vi "nanocal -- nuclear schottky fit -- 2x2 -- V9.vi"() -> ()   [LabVIEW 2021] (continued)
\"τS\" -> 0.000000000000   ,  \"τN\" -> 0.000000000000   ,  \"τC\" -> 0.000000000000   ,  \"κ0\" -> 0.000000000000   ,  \"mm1\" -> 0.000000000000   ,  \"mm2\" -> 0.000000000000   ,  \"mm3\" -> 0.000000000000   ,  \"T\" -> 3.070000000000   ,  \"B\" -> 4.000000000000   ,  \"θ\" -> 0.000000000000   ,  \"Reoff\" -> 0.000000000000   ,  \"Imoff\" -> 0.000000000000   ,  \"στ1\" -> 0.000000000000   ,  \"στS\" -> 0.000000000000   ,  \"στN\" -> 0.000000000000    |>   , \n\"IDS0473_220531_RAW_cal__ref_\" ->   <|    \"ζ\" -> 0.018700689738   ,  \"τ1\" -> 0.039247142341   ,  \"τS\" -> 0.006094502124   ,  \"τN\" -> 0.000001379348   ,  \"τC\" -> 0.001765569741   ,  \"κ0\" -> 0.000000055137   ,  \"mm1\" -> 0.000025315301   ,  \"mm2\" -> 0.007948371438   ,  \"mm3\" -> 0.039248904003   ,  \"T\" -> 5.700000000000   ,  \"B\" -> 4.000000000000   ,  \"θ\" -> 0.000000000000   ,  \"Reoff\" -> -102040.816326530650   ,  \"Imoff\" -> 0.000000000000   ,  \"στ1\" -> 0.006123782667   ,  \"στS\" -> 0.001309533453   ,  \"στN\" -> 0.000000787923    |>   , \n\"IDS0473_220531_RAW_cal__sam_\" ->   <|    \"ζ\" -> 0.000000000000   ,  \"τ1\" -> 0.000000000000   ,  \"τS\" -> 0.000000000000   ,  \"τN\" -> 0.000000000000   ,  \"τC\" -> 0.000000000000   ,  \"κ0\" -> 0.000000000000   ,  \"mm1\" -> 0.000000000000   ,  \"mm2\" -> 0.000000000000   ,  \"mm3\" -> 0.000000000000   ,  \"T\" -> 5.700000000000   ,  \"B\" -> 4.000000000000   ,  \"θ\" -> 0.000000000000   ,  \"Reoff\" -> 0.000000000000   ,  \"Imoff\" -> 0.000000000000   ,  \"στ1\" -> 0.000000000000   ,  \"στS\" -> 0.000000000000   ,  \"στN\" -> 0.000000000000    |>   , \n\"IDS0477_220601_RAW_cal__ref_\" ->   <|    \"ζ\" -> 0.239805642697   ,  \"τ1\" -> 0.033790664831   ,  \"τS\" -> 0.059024379220   ,  \"τN\" -> 0.060427064379   ,  \"τC\" -> 0.000896937980   ,  \"κ0\" -> 0.000000000920   ,  \"mm1\" -> 0.000171776345   ,  \"mm2\" -> 0.014890032084   ,  \"mm3\" -> 0.167722368184   ,  \"T\" -> 0.200000000000   ,  \"B\" -> 10.000000000000   ,  \"θ\" -> 45.000000000000   ,  \"Reoff\" -> -36122448.979591839000   ,  \"Imoff\" -> 0.000000000000   ,  \"στ1\" -> 0.011907202865   ,  \"στS\" -> 0.006392080806   ,  \"στN\" -> 0.010956766376    |>   , \n\"IDS0477_220601_RAW_cal__sam_\" ->   <|    \"ζ\" -> 0.000000000000   ,  \"τ1\" -> 0.000000000000   ,  \"τS\" -> 0.000000000000   ,  \"τN\" -> 0.000000000000   ,  \"τC\" -> 0.000000000000   ,  \"κ0\" -> 0.000000000000   ,  \"mm1\" -> 0.000000000000   ,  \"mm2\" -> 0.000000000000   ,  \"mm3\" -> 0.000000000000   ,  \"T\" -> 0.200000000000   ,  \"B\" -> 10.000000000000   ,  \"θ\" -> 45.000000000000   ,  \"Reoff\" -> 0.000000000000   ,  \"Imoff\" -> 0.000000000000   ,  \"στ1\" -> 0.000000000000   ,  \"στS\" -> 0.000000000000   ,  \"στN\" -> 0.000000000000    |>   , \n\"IDS0478_220601_RAW_cal__ref_\" ->   <|    \"ζ\" -> 0.152803180528   ,  \"τ1\" -> 0.028187868792   ,  \"τS\" -> 0.047098340694   ,  \"τN\" -> 0.025207837056   ,  \"τC\" -> 0.000982024605   ,  \"κ0\" -> 0.000000001260   ,  \"mm1\" -> 0.000128146365   ,  \"mm2\" -> 0.016152622122   ,  \"mm3\" -> 0.096243916593   ,  \"T\" -> 0.250000000000   ,  \"B\" -> 10.000000000000   ,  \"θ\" -> 45.000000000000   ,  \"Reoff\" -> -18163265.306122452000   ,  \"Imoff\" -> 0.000000000000   ,  \"στ1\" -> 0.005041045857   ,  \"στS\" -> 0.001567344139   ,  \"στN\" -> 0.002277988599    |>   , \n\"IDS0478_220601_RAW_cal__sam_\" ->   <|    \"ζ\" -> 0.000000000000   ,  \"τ1\" -> 0.000000000000   ,  \"τS\" -> 0.000000000000   ,  \"τN\" -> 0.000000000000   ,  \"τC\" -> 0.000000000000   ,  \"κ0\" -> 0.000000000000   ,  \"mm1\" -> 0.000000000000   ,  \"mm2\" -> 0.000000000000   ,  \"mm3\" -> 0.000000000000   ,  \"T\" -> 0.250000000000   ,  \"B\" -> 10.000000000000   ,  \"θ\" -> 45.000000000000   ,  \"Reoff\" -> 0.000000000000   ,  \"Imoff\" -> 0.000000000000   ,  \"στ1\" -> 0.000000000000   ,  \"στS\" -> 0.000000000000   ,  \"στN\" -> 0.000000000000    |>   , \n\"IDS0479_220601_RAW_cal__ref_\" ->   <|    \"ζ\" -> 0.111193066205   ,  \"τ1\" -> 0.024122553376   ,  \"τS\" -> 0.042118651402   ,  \"τN\" -> 0.013651970206   ,  \"τC\" -> 0.001072327817   ,  \"κ0\" -> 0.000000001570   ,  \"mm1\" -> 0.000105128315   ,  \"mm2\" -> 0.016280391263   ,  \"mm3\" -> 0.070781289644   ,  \"T\" -> 0.300000000000   ,  \"B\" -> 10.000000000000   ,  \"θ\" -> 45.000000000000   ,  \"Reoff\" -> -10816326.530612245200   ,  \"Imoff\" -> 0.000000000000   ,  \"στ1\" -> 0.003531051170   ,  \"στS\" -> 0.000678989919   ,  \"στN\" -> 0.000877996668    |>   , \n\"IDS0479_220601_RAW_cal__sam_\" ->   <|    \"ζ\" -> 0.000000000000   ,  \"τ1\" -> 0.000000000000   ,  \"τS\" -> 0.000000000000   ,  \"τN\" -> 0.000000000000   ,  \"τC\" -> 0.000000000000   ,  \"κ0\" -> 0.000000000000   ,  \"mm1\" -> 0.000000000000   ,  \"mm2\" -> 0.000000000000   ,  \"mm3\" -> 0.000000000000   ,  \"T\" -> 0.300000000000   ,  \"B\" -> 10.000000000000   ,  \"θ\" -> 45.000000000000   ,  \"Reoff\" -> 0.000000000000   ,  \"Imoff\" -> 0.000000000000   ,  \"στ1\" -> 0.000000000000   ,  \"στS\" -> 0.000000000000   ,  \"στN\" -> 0.000000000000    |>   , \n\"IDS0480_220601_RAW_cal__ref_\" ->   <|    \"ζ\" -> 0.079231560459   ,  \"τ1\" -> 0.017107381840   ,  \"τS\" -> 0.036891145607   ,  \"τN\" -> 0.007202328301   ,  \"τC\" -> 0.001264563258   ,  \"κ0\" -> 0.000000002000   ,  \"mm1\" -> 0.000090175019   ,  \"mm2\" -> 0.013352548983   ,  \"mm3\" -> 0.052516289748   ,  \"T\" -> 0.360000000000   ,  \"B\" -> 10.000000000000   ,  \"θ\" -> 45.000000000000   ,  \"Reoff\" -> -6326530.612244904040   ,  \"Imoff\" -> 0.000000000000   ,  \"στ1\" -> 0.001933309697   ,  \"στS\" -> 0.000284795622   ,  \"στN\" -> 0.000344056722    |>   , \n\"IDS0480_220601_RAW_cal__sam_\" ->   <|    \"ζ\" -> 0.000000000000   ,  \"τ1\" -> 0.000000000000   ,  \"τS\" -> 0.000000000000   ,  \"τN\" -> 0.000000000000   ,  \"τC\" -> 0.000000000000   ,  \"κ0\" -> 0.000000000000   ,  \"mm1\" -> 0.000000000000   ,  \"mm2\" -> 0.000000000000   ,  \"mm3\" -> 0.000000000000   ,  \"T\" -> 0.360000000000   ,  \"B\" -> 10.000000000000   ,  \"θ\" -> 45.000000000000   ,  \"Reoff\" -> 0.000000000000   ,  \"Imoff\" -> 0.000000000000   ,  \"στ1\" -> 0.000000000000   ,  \"στS\" -> 0.000000000000   ,  \"στN\" -> 0.000000000000    |>   , \n\"IDS0481_220601_RAW_cal__ref_\" ->   <|    \"ζ\" -> 0.059346185114   ,  \"τ1\" -> 0.015969775027   ,  \"τS\" -> 0.034144098652   ,  \"τN\" -> 0.004294468384   ,  \"τC\" -> 0.001604549811   ,  \"κ0\" -> 0.000000002410   ,  \"mm1\" -> 0.000086265768   ,  \"mm2\" -> 0.013446939913   ,  \"mm3\" -> 0.044760868507   ,  \"T\" -> 0.420000000000   ,  \"B\" -> 10.000000000000   ,  \"θ\" -> 45.000000000000   ,  \"Reoff\" -> -3061224.489795923230   ,  \"Imoff\" -> 0.000000000000   ,  \"στ1\" -> 0.000907344416   ,  \"στS\" -> 0.000176030005   ,  \"στN\" -> 0.000148751487    |>   , \n\"IDS0481_220601_RAW_cal__sam_\" ->   <|    \"ζ\" -> 0.000000000000   ,  \"τ1\" -> 0.000000000000   ,  \"τS\" -> 0.000000000000   ,  \"τN\" -> 0.000000000000   ,  \"τC\" -> 0.000000000000   ,  \"κ0\" -> 0.000000000000   ,  \"mm1\" -> 0.000000000000   ,  \"mm2\" -> 0.000000000000   ,  \"mm3\" -> 0.000000000000   ,  \"T\" -> 0.420000000000   ,  \"B\" -> 10.000000000000   ,  \"θ\" -> 45.000000000000   ,  \"Reoff\" -> 0.000000000000   ,  \"Imoff\" -> 0.000000000000   ,  \"στ1\" -> 0.000000000000   ,  \"στS\" -> 0.000000000000   ,  \"στN\" -> 0.000000000000    |>   , \n\"IDS0482_220601_RAW_cal__ref_\" ->   <|    \"ζ\" -> 0.043142553496   ,  \"τ1\" -> 0.014499389185   ,  \"τS\" -> 0.030371945733   ,  \"τN\" -> 0.002402650316   ,  \"τC\" -> 0.001877907190   ,  \"κ0\" -> 0.000000003100   ,  \"mm1\" -> 0.000073480289   ,  \"mm2\" -> 0.012924539137   ,  \"mm3\" -> 0.037567852762   ,  \"T\" -> 0.520000000000   ,  \"B\" -> 10.000000000000   ,  \"θ\" -> 45.000000000000   ,  \"Reoff\" -> -1836734.693877555430   ,  \"Imoff\" -> 0.000000000000   ,  \"στ1\" -> 0.000488095502   ,  \"στS\" -> 0.000097405917   ,  \"στN\" -> 0.000051506778    |>   , \n\"IDS0482_220601_RAW_cal__sam_\" ->   <|    \"ζ\" -> 0.000000000000   ,  \"τ1\" -> 0.000000000000   ,  \"τS\" -> 0.000000000000   ,  \"τN\" -> 0.000000000000   ,  \"τC\" -> 0.000000000000   ,  \"κ0\" -> 0.000000000000   ,  \"mm1\" -> 0.000000000000   ,  \"mm2\" -> 0.000000000000   ,  \"mm3\" -> 0.000000000000   ,  \"T\" -> 0.520000000000   ,  \"B\" -> 10.000000000000   ,  \"θ\" -> 45.000000000000   ,  \"Reoff\" -> 0.000000000000   ,  \"Imoff\" -> 0.000000000000   ,  \"στ1\" -> 0.000000000000   ,  \"στS\" -> 0.000000000000   ,  \"στN\" -> 0.000000000000    |>   , \n\"IDS0483_220601_RAW_cal__ref_\" ->   <|    \"ζ\" -> 0.037957534412   ,  \"τ1\" -> 0.013025982486   ,  \"τS\" -> 0.027861955043   ,  \"τN\" -> 0.001482537125   ,  \"τC\" -> 0.001562153050   ,  \"κ0\" -> 0.000000003750   ,  \"mm1\" -> 0.000054295490   ,  \"mm2\" -> 0.012021211304   ,  \"mm3\" -> 0.032970965481   ,  \"T\" -> 0.620000000000   ,  \"B\" -> 10.000000000000   ,  \"θ\" -> 45.000000000000   ,  \"Reoff\" -> -2489795.918367348610   ,  \"Imoff\" -> 0.000000000000   ,  \"στ1\" -> 0.000872811735   ,  \"στS\" -> 0.000114206450   ,  \"στN\" -> 0.000055407234    |>   , \n\"IDS0483_220601_RAW_cal__sam_\" ->   <|    \"ζ\" -> 0.000000000000   ,  \"τ1\" -> 0.000000000000   ,  \"τS\" -> 0.000000000000   ,  \"τN\" -> 0.000000000000   ,  \"τC\" -> 0.000000000000   ,  \"κ0\" -> 0.000000000000   ,  \"mm1\" -> 0.000000000000   ,  \"mm2\" -> 0.000000000000   ,  \"mm3\" -> 0.000000000000   ,  \"T\" -> 0.620000000000   ,  \"B\" -> 10.000000000000   ,  \"θ\" -> 45.000000000000   ,  \"Reoff\" -> 0.000000000000   ,  \"Imoff\" -> 0.000000000000   ,  \"στ1\" -> 0.000000000000   ,  \"στS\" -> 0.000000000000   ,  \"στN\" -> 0.000000000000    |>   , \n\"IDS0484_220601_RAW_cal__ref_\" ->   <|    \"ζ\" -> 0.026779879048   ,  \"τ1\" -> 0.012724854717   ,  \"τS\" -> 0.023406495826   ,  \"τN\" -> 0.000845574693   ,  \"τC\" -> 0.002190018434   ,  \"κ0\" -> 0.000000005114   ,  \"mm1\" -> 0.000052452848   ,  \"mm2\" -> 0.011990951083   ,  \"mm3\" -> 0.027773007254   ,  \"T\" -> 0.820000000000   ,  \"B\" -> 10.000000000000   ,  \"θ\" -> 45.000000000000   ,  \"Reoff\" -> -1020408.163265310230   ,  \"Imoff\" -> 0.000000000000   ,  \"στ1\" -> 0.000585844678   ,  \"στS\" -> 0.000123901377   ,  \"στN\" -> 0.000022627070    |>   , \n\"IDS0484_220601_RAW_cal__sam_\" ->   <|    \"ζ\" -> 0.000000000000   ,  \"τ1\" -> 0.000000000000   ,  \"τS\" -> 0.000000000000   ,  \"τN\" -> 0.000000000000   ,  \"τC\" -> 0.000000000000   ,  \"κ0\" -> 0.000000000000   ,  \"mm1\" -> 0.000000000000   ,  \"mm2\" -> 0.000000000000   ,  \"mm3\" -> 0.000000000000   ,  \"T\" -> 0.820000000000   ,  \"B\" -> 10.000000000000   ,  \"θ\" -> 45.000000000000   ,  \"Reoff\" -> 0.000000000000   ,  \"Imoff\" -> 0.000000000000   ,  \"στ1\" -> 0.000000000000   ,  \"στS\" -> 0.000000000000   ,  \"στN\" -> 0.000000000000    |>   , \n\"IDS0485_220601_RAW_cal__ref_\" ->   <|    \"ζ\" -> 0.326622885443   ,  \"τ1\" -> 0.044212332753   ,  \"τS\" -> 0.078119393187   ,  \"τN\" -> 0.109436103453   ,  \"τC\" -> 0.000856629079   ,  \"κ0\" -> 0.000000000725   ,  \"mm1\" -> 0.000209590105   ,  \"mm2\" -> 0.016643396508   ,  \"mm3\" -> 0.277031389353   ,  \"T\" -> 0.170000000000   ,  \"B\" -> 10.000000000000   ,  \"θ\" -> 45.000000000000   ,  \"Reoff\" -> -62040816.326530613000   ,  \"Imoff\" -> 0.000000000000   ,  \"στ1\" -> 0.024054965225   ,  \"στS\" -> 0.017110063636   ,  \"στN\" -> 0.032486922745    |>   , \n\"IDS0485_220601_RAW_cal__sam_\" ->   <|    \"ζ\" -> 0.000000000000   ,  \"τ1\" -> 0.000000000000   ,  \"τS\" -> 0.000000000000   ,  \"τN\" -> 0.000000000000   ,  \"τC\" -> 0.000000000000   ,  \"κ0\" -> 0.000000000000   ,  \"mm1\" -> 0.000000000000   ,  \"mm2\" -> 0.000000000000   ,  \"mm3\" -> 0.000000000000   ,  \"T\" -> 0.170000000000   ,  \"B\" -> 10.000000000000   ,  \"θ\" -> 45.000000000000   ,  \"Reoff\" -> 0.000000000000   ,  \"Imoff\" -> 0.000000000000   ,  \"στ1\" -> 0.000000000000   ,  \"στS\" -> 0.000000000000   ,  \"στN\" -> 0.000000000000    |>   , \n\"IDS0486_220602_RAW_cal__ref_\" ->   <|    \"ζ\" -> 0.647357967210   ,  \"τ1\" -> 0.057848718155   ,  \"τS\" -> 0.135216834392   ,  \"τN\" -> 0.439833290844   ,  \"τC\" -> 0.000803496040   ,  \"κ0\" -> 0.000000000457   ,  \"mm1\" -> 0.000315044381   ,  \"mm2\" -> 0.013010354662   ,  \"mm3\" -> 0.992640220504   ,  \"T\" -> 0.120000000000   ,  \"B\" -> 10.000000000000   ,  \"θ\" -> 45.000000000000   ,  \"Reoff\" -> -171836734.693877578000   ,  \"Imoff\" -> 0.000000000000   ,  \"στ1\" -> 0.042149570105   ,  \"στS\" -> 0.062954836972   ,  \"στN\" -> 0.160749966190    |>   , \n\"IDS0486_220602_RAW_cal__sam_\" ->   <|    \"ζ\" -> 0.000000000000   ,  \"τ1\" -> 0.000000000000   ,  \"τS\" -> 0.000000000000   ,  \"τN\" -> 0.000000000000   ,  \"τC\" -> 0.000000000000   ,  \"κ0\" -> 0.000000000000   ,  \"mm1\" -> 0.000000000000   ,  \"mm2\" -> 0.000000000000   ,  \"mm3\" -> 0.000000000000   ,  \"T\" -> 0.120000000000   ,  \"B\" -> 10.000000000000   ,  \"θ\" -> 45.000000000000   ,  \"Reoff\" -> 0.000000000000   ,  \"Imoff\" -> 0.000000000000   ,  \"στ1\" -> 0.000000000000   ,  \"στS\" -> 0.000000000000   ,  \"στN\" -> 0.000000000000    |>   , \n\"IDS0487_220602_RAW_cal__ref_\" ->   <|    \"ζ\" -> 0.413977366659   ,  \"τ1\" -> 0.044491025512   ,  \"τS\" -> 0.091456784931   ,  \"τN\" -> 0.162770283044   ,  \"τC\" -> 0.000783758784   ,  \"κ0\" -> 0.000000000637   ,  \"mm1\" -> 0.000228474902   ,  \"mm2\" -> 0.014828264072   ,  \"mm3\" -> 0.389689365431   ,  \"T\" -> 0.150000000000   ,  \"B\" -> 10.000000000000   ,  \"θ\" -> 45.000000000000   ,  \"Reoff\" -> -87632653.061224490400   ,  \"Imoff\" -> 0.000000000000   ,  \"στ1\" -> 0.020687994730   ,  \"στS\" -> 0.021344943576   ,  \"στN\" -> 0.040787910782    |>   , \n\"IDS0487_220602_RAW_cal__sam_\" ->   <|    \"ζ\" -> 0.000000000000   ,  \"τ1\" -> 0.000000000000   ,  \"τS\" -> 0.000000000000   ,  \"τN\" -> 0.000000000000   ,  \"τC\" -> 0.000000000000   ,  \"κ0\" -> 0.000000000000   ,  \"mm1\" -> 0.000000000000   ,  \"mm2\" -> 0.000000000000   ,  \"mm3\" -> 0.000000000000   ,  \"T\" -> 0.150000000000   ,  \"B\" -> 10.000000000000   ,  \"θ\" -> 45.000000000000   ,  \"Reoff\" -> 0.000000000000   ,  \"Imoff\" -> 0.000000000000   ,  \"στ1\" -> 0.000000000000   ,  \"στS\" -> 0.000000000000   ,  \"στN\" -> 0.000000000000    |>   , \n\"IDS0488_220602_RAW_cal__ref_\" ->   <|    \"ζ\" -> 0.022173506919   ,  \"τ1\" -> 0.011885040231   ,  \"τS\" -> 0.019213986471   ,  \"τN\" -> 0.000342476634   ,  \"τC\" -> 0.002250605678   ,  \"κ0\" -> 0.000000007250   ,  \"mm1\" -> 0.000043889604   ,  \"mm2\" -> 0.011496376729   ,  \"mm3\" -> 0.022585478052   ,  \"T\" -> 1.120000000000   ,  \"B\" -> 10.000000000000   ,  \"θ\" -> 45.000000000000   ,  \"Reoff\" -> -775510.204081632196   ,  \"Imoff\" -> 0.000000000000   ,  \"στ1\" -> 0.000592033773   ,  \"στS\" -> 0.000127596201   ,  \"στN\" -> 0.000006161863    |>   , \n\"IDS0488_220602_RAW_cal__sam_\" ->   <|    \"ζ\" -> 0.000000000000   ,  \"τ1\" -> 0.000000000000   ,  \"τS\" -> 0.000000000000   ,  \"τN\" -> 0.000000000000   ,  \"τC\" -> 0.000000000000   ,  \"κ0\" -> 0.000000000000   ,  \"mm1\" -> 0.000000000000   ,  \"mm2\" -> 0.000000000000   ,  \"mm3\" -> 0.000000000000   ,  \"T\" -> 1.120000000000   ,  \"B\" -> 10.000000000000   ,  \"θ\" -> 45.000000000000   ,  \"Reoff\" -> 0.000000000000   ,  \"Imoff\" -> 0.000000000000   ,  \"στ1\" -> 0.000000000000   ,  \"στS\" -> 0.000000000000   ,  \"στN\" -> 0.000000000000    |>   , \n\"IDS0489_220602_RAW_cal__ref_\" ->   <|    \"ζ\" -> 0.017747577510   ,  \"τ1\" -> 0.012094843134   ,  \"τS\" -> 0.012989013001   ,  \"τN\" -> 0.000085603032   ,  \"τC\" -> 0.003089605627   ,  \"κ0\" -> 0.000000012681   ,  \"mm1\" -> 0.000043787767   ,  \"mm2\" -> 0.011860461021   ,  \"mm3\" -> 0.016586858767   ,  \"T\" -> 1.900000000000   ,  \"B\" -> 10.000000000000   ,  \"θ\" -> 45.000000000000   ,  \"Reoff\" -> -285714.285714283585   ,  \"Imoff\" -> 0.000000000000   ,  \"στ1\" -> 0.000492222129   ,  \"στS\" -> 0.000068169784   ,  \"στN\" -> 0.000002379689    |>   , \n\"IDS0489_220602_RAW_cal__sam_\" ->   <|    \"ζ\" -> 0.000000000000   ,  \"τ1\" -> 0.000000000000   ,  \"τS\" -> 0.000000000000   ,  \"τN\" -> 0.000000000000   ,  \"τC\" -> 0.000000000000   ,  \"κ0\" -> 0.000000000000   ,  \"mm1\" -> 0.000000000000   ,  \"mm2\" -> 0.000000000000   ,  \"mm3\" -> 0.000000000000   ,  \"T\" -> 1.900000000000   ,  \"B\" -> 10.000000000000   ,  \"θ\" -> 45.000000000000   ,  \"Reoff\" -> 0.000000000000   ,  \"Imoff\" -> 0.000000000000   ,  \"στ1\" -> 0.000000000000   ,  \"στS\" -> 0.000000000000   ,  \"στN\" -> 0.000000000000    |>   , \n\"IDS0490_220602_RAW_cal__ref_\" ->   <|    \"ζ\" -> 0.017719366864   ,  \"τ1\" -> 0.012304843107   ,  \"τS\" -> 0.009230373075   ,  \"τN\" -> 0.000023645241   ,  \"τC\" -> 0.002722388049   ,  \"κ0\" -> 0.000000022572   ,  \"mm1\" -> 0.000036861190   ,  \"mm2\" -> 0.011651022890   ,  \"mm3\" -> 0.012757340738   ,  \"T\" -> 3.100000000000   ,  \"B\" -> 10.000000000000   ,  \"θ\" -> 45.000000000000   ,  \"Reoff\" -> -204081.632653061300   ,  \"Imoff\" -> 0.000000000000   ,  \"στ1\" -> 0.000238275245   ,  \"στS\" -> 0.000083164391   ,  \"στN\" -> 0.000000428704    |>   , \n\"IDS0490_220602_RAW_cal__sam_\" ->   <|    \"ζ\" -> 0.000000000000   ,  \"τ1\" -> 0.000000000000   ,  \"τS\" -> 0.000000000000   ,  \"τN\" -> 0.000000000000   ,  \"τC\" -> 0.000000000000   ,  \"κ0\" -> 0.000000000000   ,  \"mm1\" -> 0.000000000000   ,  \"mm2\" -> 0.000000000000   ,  \"mm3\" -> 0.000000000000   ,  \"T\" -> 3.100000000000   ,  \"B\" -> 10.000000000000   ,  \"θ\" -> 45.000000000000   ,  \"Reoff\" -> 0.000000000000   ,  \"Imoff\" -> 0.000000000000   ,  \"στ1\" -> 0.000000000000   ,  \"στS\" -> 0.000000000000   ,  \"στN\" -> 0.000000000000    |>   , \n\"IDS0491_220602_RAW_cal__ref_\" ->   <|    \"ζ\" -> 0.018539000460   ,  \"τ1\" -> 0.012513981678   ,  \"τS\" -> 0.005770088680   ,  \"τN\" -> 0.000004734838   ,  \"τC\" -> 0.002222689414   ,  \"κ0\" -> 0.000000055495   ,  \"mm1\" -> 0.000029461735   ,  \"mm2\" -> 0.008061568111   ,  \"mm3\" -> 0.012527524219   ,  \"T\" -> 5.700000000000   ,  \"B\" -> 10.000000000000   ,  \"θ\" -> 45.000000000000   ,  \"Reoff\" -> -69387.755102040828   ,  \"Imoff\" -> 0.000000000000   ,  \"στ1\" -> 0.001996888534   ,  \"στS\" -> 0.001027587268   ,  \"στN\" -> 0.000002006873    |>   , \n\"IDS0491_220602_RAW_cal__sam_\" ->   <|    \"ζ\" -> 0.000000000000   ,  \"τ1\" -> 0.000000000000   ,  \"τS\" -> 0.000000000000   ,  \"τN\" -> 0.000000000000   ,  \"τC\" -> 0.000000000000   ,  \"κ0\" -> 0.000000000000   ,  \"mm1\" -> 0.000000000000   ,  \"mm2\" -> 0.000000000000   ,  \"mm3\" -> 0.000000000000   ,  \"T\" -> 5.700000000000   ,  \"B\" -> 10.000000000000   ,  \"θ\" -> 45.000000000000   ,  \"Reoff\" -> 0.000000000000   ,  \"Imoff\" -> 0.000000000000   ,  \"στ1\" -> 0.000000000000   ,  \"στS\" -> 0.000000000000   ,  \"στN\" -> 0.000000000000    |>   , \n\"IDS0493_220602_RAW_cal__ref_\" ->   <|    \"ζ\" -> 0.240316518824   ,  \"τ1\" -> 0.030134211391   ,  \"τS\" -> 0.077333506670   ,  \"τN\" -> 0.032228870252   ,  \"τC\" -> 0.000888040946   ,  \"κ0\" -> 0.000000000940   ,  \"mm1\" -> 0.000170781534   ,  \"mm2\" -> 0.019820439561   ,  \"mm3\" -> 0.146923057180   ,  \"T\" -> 0.200000000000   ,  \"B\" -> 8.000000000000   ,  \"θ\" -> 45.000000000000   ,  \"Reoff\" -> -33763265.306122481800   ,  \"Imoff\" -> 0.000000000000   ,  \"στ1\" -> 0.022409669919   ,  \"στS\" -> 0.010038141046   ,  \"στN\" -> 0.010969652299    |>   , \n\"IDS0493_220602_RAW_cal__sam_\" ->   <|    \"ζ\" -> 0.000000000000   ,  \"τ1\" -> 0.000000000000   ,  \"τS\" -> 0.000000000000   ,  \"τN\" -> 0.000000000000   ,  \"τC\" -> 0.000000000000   ,  \"κ0\" -> 0.000000000000   ,  \"mm1\" -> 0.000000000000   ,  \"mm2\" -> 0.000000000000   ,  \"mm3\" -> 0.000000000000   ,  \"T\" -> 0.200000000000   ,  \"B\" -> 8.000000000000   ,  \"θ\" -> 45.000000000000   ,  \"Reoff\" -> 0.000000000000   ,  \"Imoff\" -> 0.000000000000   ,  \"στ1\" -> 0.000000000000   ,  \"στS\" -> 0.000000000000   ,  \"στN\" -> 0.000000000000    |>   , \n\"IDS0494_220602_RAW_cal__ref_\" ->   <|    \"ζ\" -> 0.158252879790   ,  \"τ1\" -> 0.024827950008   ,  \"τS\" -> 0.060146890842   ,  \"τN\" -> 0.015050943013   ,  \"τC\" -> 0.000951750255   ,  \"κ0\" -> 0.000000001243   ,  \"mm1\" -> 0.000128517617   ,  \"mm2\" -> 0.018585917114   ,  \"mm3\" -> 0.094163373149   ,  \"T\" -> 0.250000000000   ,  \"B\" -> 8.000000000000   ,  \"θ\" -> 45.000000000000   ,  \"Reoff\" -> -20024489.795918367800   ,  \"Imoff\" -> 0.000000000000   ,  \"στ1\" -> 0.008614865267   ,  \"στS\" -> 0.002364789587   ,  \"στN\" -> 0.002490160339    |>   , \n\"IDS0494_220602_RAW_cal__sam_\" ->   <|    \"ζ\" -> 0.000000000000   ,  \"τ1\" -> 0.000000000000   ,  \"τS\" -> 0.000000000000   ,  \"τN\" -> 0.000000000000   ,  \"τC\" -> 0.000000000000   ,  \"κ0\" -> 0.000000000000   ,  \"mm1\" -> 0.000000000000   ,  \"mm2\" -> 0.000000000000   ,  \"mm3\" -> 0.000000000000   ,  \"T\" -> 0.250000000000   ,  \"B\" -> 8.000000000000   ,  \"θ\" -> 45.000000000000   ,  \"Reoff\" -> 0.000000000000   ,  \"Imoff\" -> 0.000000000000   ,  \"στ1\" -> 0.000000000000   ,  \"στS\" -> 0.000000000000   ,  \"στN\" -> 0.000000000000    |>   , \n\"IDS0495_220602_RAW_cal__ref_\" ->   <|    \"ζ\" -> 0.620326639374   ,  \"τ1\" -> 0.043464597459   ,  \"τS\" -> 0.134106398601   ,  \"τN\" -> 0.331630286291   ,  \"τC\" -> 0.000791545838   ,  \"κ0\" -> 0.000000000449   ,  \"mm1\" -> 0.000302343125   ,  \"mm2\" -> 0.012035033998   ,  \"mm3\" -> 0.786564323638   ,  \"T\" -> 0.120000000000   ,  \"B\" -> 8.000000000000   ,  \"θ\" -> 45.000000000000   ,  \"Reoff\" -> -197355102.040816367000   ,  \"Imoff\" -> 0.000000000000   ,  \"στ1\" -> 0.040479747535   ,  \"στS\" -> 0.067583774677   ,  \"στN\" -> 0.126300079114    |>   , \n\"IDS0495_220602_RAW_cal__sam_\" ->   <|    \"ζ\" -> 0.000000000000   ,  \"τ1\" -> 0.000000000000   ,  \"τS\" -> 0.000000000000   ,  \"τN\" -> 0.000000000000   ,  \"τC\" -> 0.000000000000   ,  \"κ0\" -> 0.000000000000   ,  \"mm1\" -> 0.000000000000   ,  \"mm2\" -> 0.000000000000   ,  \"mm3\" -> 0.000000000000   ,  \"T\" -> 0.120000000000   ,  \"B\" -> 8.000000000000   ,  \"θ\" -> 45.000000000000   ,  \"Reoff\" -> 0.000000000000   ,  \"Imoff\" -> 0.000000000000   ,  \"στ1\" -> 0.000000000000   ,  \"στS\" -> 0.000000000000   ,  \"στN\" -> 0.000000000000    |>   , \n\"IDS0496_220602_RAW_cal__ref_\" ->   <|    \"ζ\" -> 0.427468854343   ,  \"τ1\" -> 0.039705721457   ,  \"τS\" -> 0.111520336177   ,  \"τN\" -> 0.118737423491   ,  \"τC\" -> 0.000757643682   ,  \"κ0\" -> 0.000000000613   ,  \"mm1\" -> 0.000226123834   ,  \"mm2\" -> 0.018076446652   ,  \"mm3\" -> 0.350846575050   ,  \"T\" -> 0.150000000000   ,  \"B\" -> 8.000000000000   ,  \"θ\" -> 45.000000000000   ,  \"Reoff\" -> -103289795.918367386000   ,  \"Imoff\" -> 0.000000000000   ,  \"στ1\" -> 0.024554050195   ,  \"στS\" -> 0.027075430846   ,  \"στN\" -> 0.033199054106    |>   , \n\"IDS0496_220602_RAW_cal__sam_\" ->   <|    \"ζ\" -> 0.000000000000   ,  \"τ1\" -> 0.000000000000   ,  \"τS\" -> 0.000000000000   ,  \"τN\" -> 0.000000000000   ,  \"τC\" -> 0.000000000000   ,  \"κ0\" -> 0.000000000000   ,  \"mm1\" -> 0.000000000000   ,  \"mm2\" -> 0.000000000000   ,  \"mm3\" -> 0.000000000000   ,  \"T\" -> 0.150000000000   ,  \"B\" -> 8.000000000000   ,  \"θ\" -> 45.000000000000   ,  \"Reoff\" -> 0.000000000000   ,  \"Imoff\" -> 0.000000000000   ,  \"στ1\" -> 0.000000000000   ,  \"στS\" -> 0.000000000000   ,  \"στN\" -> 0.000000000000    |>   , \n\"IDS0497_220603_RAW_cal__ref_\" ->   <|    \"ζ\" -> 0.332403347952   ,  \"τ1\" -> 0.033892588666   ,  \"τS\" -> 0.089882476524   ,  \"τN\" -> 0.072116867912   ,  \"τC\" -> 0.000736636997   ,  \"κ0\" -> 0.000000000736   ,  \"mm1\" -> 0.000182924179   ,  \"mm2\" -> 0.017518148856   ,  \"mm3\" -> 0.232776621520   ,  \"T\" -> 0.170000000000   ,  \"B\" -> 8.000000000000   ,  \"θ\" -> 45.000000000000   ,  \"Reoff\" -> -72616326.530612289900   ,  \"Imoff\" -> 0.000000000000   ,  \"στ1\" -> 0.010864544003   ,  \"στS\" -> 0.009543194360   ,  \"στN\" -> 0.010830263954    |>   , \n\"IDS0497_220603_RAW_cal__sam_\" ->   <|    \"ζ\" -> 0.000000000000   ,  \"τ1\" -> 0.000000000000   ,  \"τS\" -> 0.000000000000   ,  \"τN\" -> 0.000000000000   ,  \"τC\" -> 0.000000000000   ,  \"κ0\" -> 0.000000000000   ,  \"mm1\" -> 0.000000000000   ,  \"mm2\" -> 0.000000000000   ,  \"mm3\" -> 0.000000000000   ,  \"T\" -> 0.170000000000   ,  \"B\" -> 8.000000000000   ,  \"θ\" -> 45.000000000000   ,  \"Reoff\" -> 0.000000000000   ,  \"Imoff\" -> 0.000000000000   ,  \"στ1\" -> 0.000000000000   ,  \"στS\" -> 0.000000000000   ,  \"στN\" -> 0.000000000000    |>   , \n\"IDS0498_220603_RAW_cal__ref_\" ->   <|    \"ζ\" -> 0.110734162984   ,  \"τ1\" -> 0.019381596449   ,  \"τS\" -> 0.049800010244   ,  \"τN\" -> 0.007874153241   ,  \"τC\" -> 0.001094666009   ,  \"κ0\" -> 0.000000001580   ,  \"mm1\" -> 0.000107216591   ,  \"mm2\" -> 0.015930752272   ,  \"mm3\" -> 0.068498957299   ,  \"T\" -> 0.300000000000   ,  \"B\" -> 8.000000000000   ,  \"θ\" -> 45.000000000000   ,  \"Reoff\" -> -10657142.857142858200   ,  \"Imoff\" -> 0.000000000000   ,  \"στ1\" -> 0.007394501349   ,  \"στS\" -> 0.001744107422   ,  \"στN\" -> 0.001987690041    |>   , \n\"IDS0498_220603_RAW_cal__sam_\" ->   <|    \"ζ\" -> 0.000000000000   ,  \"τ1\" -> 0.000000000000   ,  \"τS\" -> 0.000000000000   ,  \"τN\" -> 0.000000000000   ,  \"τC\" -> 0.000000000000   ,  \"κ0\" -> 0.000000000000   ,  \"mm1\" -> 0.000000000000   ,  \"mm2\" -> 0.000000000000   ,  \"mm3\" -> 0.000000000000   ,  \"T\" -> 0.300000000000   ,  \"B\" -> 8.000000000000   ,  \"θ\" -> 45.000000000000   ,  \"Reoff\" -> 0.000000000000   ,  \"Imoff\" -> 0.000000000000   ,  \"στ1\" -> 0.000000000000   ,  \"στS\" -> 0.000000000000   ,  \"στN\" -> 0.000000000000    |>   , \n\"IDS0499_220603_RAW_cal__ref_\" ->   <|    \"ζ\" -> 0.075729964973   ,  \"τ1\" -> 0.017492157350   ,  \"τS\" -> 0.042916924435   ,  \"τN\" -> 0.003910009488   ,  \"τC\" -> 0.001485143735   ,  \"κ0\" -> 0.000000001996   ,  \"mm1\" -> 0.000101508308   ,  \"mm2\" -> 0.015465208626   ,  \"mm3\" -> 0.053783720140   ,  \"T\" -> 0.360000000000   ,  \"B\" -> 8.000000000000   ,  \"θ\" -> 45.000000000000   ,  \"Reoff\" -> -3787755.102040812380   ,  \"Imoff\" -> 0.000000000000   ,  \"στ1\" -> 0.001180089795   ,  \"στS\" -> 0.000447730504   ,  \"στN\" -> 0.000150733035    |>   , \n\"IDS0499_220603_RAW_cal__sam_\" ->   <|    \"ζ\" -> 0.000000000000   ,  \"τ1\" -> 0.000000000000   ,  \"τS\" -> 0.000000000000   ,  \"τN\" -> 0.000000000000   ,  \"τC\" -> 0.000000000000   ,  \"κ0\" -> 0.000000000000   ,  \"mm1\" -> 0.000000000000   ,  \"mm2\" -> 0.000000000000   ,  \"mm3\" -> 0.000000000000   ,  \"T\" -> 0.360000000000   ,  \"B\" -> 8.000000000000   ,  \"θ\" -> 45.000000000000   ,  \"Reoff\" -> 0.000000000000   ,  \"Imoff\" -> 0.000000000000   ,  \"στ1\" -> 0.000000000000   ,  \"στS\" -> 0.000000000000   ,  \"στN\" -> 0.000000000000    |>   , \n\"IDS0500_220603_RAW_cal__ref_\" ->   <|    \"ζ\" -> 0.057062025730   ,  \"τ1\" -> 0.015621328716   ,  \"τS\" -> 0.037684759429   ,  \"τN\" -> 0.002528358408   ,  \"τC\" -> 0.001814587656   ,  \"κ0\" -> 0.000000002409   ,  \"mm1\" -> 0.000093897005   ,  \"mm2\" -> 0.014229954054   ,  \"mm3\" -> 0.045619825114   ,  \"T\" -> 0.420000000000   ,  \"B\" -> 8.000000000000   ,  \"θ\" -> 45.000000000000   ,  \"Reoff\" -> -1914285.714285716420   ,  \"Imoff\" -> 0.000000000000   ,  \"στ1\" -> 0.000955516526   ,  \"στS\" -> 0.000234895501   ,  \"στN\" -> 0.000135281330    |>   , \n\"IDS0500_220603_RAW_cal__sam_\" ->   <|    \"ζ\" -> 0.000000000000   ,  \"τ1\" -> 0.000000000000   ,  \"τS\" -> 0.000000000000   ,  \"τN\" -> 0.000000000000   ,  \"τC\" -> 0.000000000000   ,  \"κ0\" -> 0.000000000000   ,  \"mm1\" -> 0.000000000000   ,  \"mm2\" -> 0.000000000000   ,  \"mm3\" -> 0.000000000000   ,  \"T\" -> 0.420000000000   ,  \"B\" -> 8.000000000000   ,  \"θ\" -> 45.000000000000   ,  \"Reoff\" -> 0.000000000000   ,  \"Imoff\" -> 0.000000000000   ,  \"στ1\" -> 0.000000000000   ,  \"στS\" -> 0.000000000000   ,  \"στN\" -> 0.000000000000    |>   , \n\"IDS0501_220603_RAW_cal__ref_\" ->   <|    \"ζ\" -> 0.041820610943   ,  \"τ1\" -> 0.014727705147   ,  \"τS\" -> 0.032103066270   ,  \"τN\" -> 0.001402697929   ,  \"τC\" -> 0.002062288671   ,  \"κ0\" -> 0.000000003070   ,  \"mm1\" -> 0.000078146988   ,  \"mm2\" -> 0.013796091461   ,  \"mm3\" -> 0.037822751096   ,  \"T\" -> 0.520000000000   ,  \"B\" -> 8.000000000000   ,  \"θ\" -> 45.000000000000   ,  \"Reoff\" -> -1155102.040816326160   ,  \"Imoff\" -> 0.000000000000   ,  \"στ1\" -> 0.000294282186   ,  \"στS\" -> 0.000104705305   ,  \"στN\" -> 0.000024302938    |>   , \n\"IDS0501_220603_RAW_cal__sam_\" ->   <|    \"ζ\" -> 0.000000000000   ,  \"τ1\" -> 0.000000000000   ,  \"τS\" -> 0.000000000000   ,  \"τN\" -> 0.000000000000   ,  \"τC\" -> 0.000000000000   ,  \"κ0\" -> 0.000000000000   ,  \"mm1\" -> 0.000000000000   ,  \"mm2\" -> 0.000000000000   ,  \"mm3\" -> 0.000000000000   ,  \"T\" -> 0.520000000000   ,  \"B\" -> 8.000000000000   ,  \"θ\" -> 45.000000000000   ,  \"Reoff\" -> 0.000000000000   ,  \"Imoff\" -> 0.000000000000   ,  \"στ1\" -> 0.000000000000   ,  \"στS\" -> 0.000000000000   ,  \"στN\" -> 0.000000000000    |>   , \n\"IDS0502_220603_RAW_cal__ref_\" ->   <|    \"ζ\" -> 0.034670986979   ,  \"τ1\" -> 0.014178027620   ,  \"τS\" -> 0.028243061757   ,  \"τN\" -> 0.000956770293   ,  \"τC\" -> 0.002118106957   ,  \"κ0\" -> 0.000000003766   ,  \"mm1\" -> 0.000066318852   ,  \"mm2\" -> 0.013432939767   ,  \"mm3\" -> 0.033009095005   ,  \"T\" -> 0.620000000000   ,  \"B\" -> 8.000000000000   ,  \"θ\" -> 45.000000000000   ,  \"Reoff\" -> -1228571.428571428170   ,  \"Imoff\" -> 0.000000000000   ,  \"στ1\" -> 0.000460475840   ,  \"στS\" -> 0.000103102463   ,  \"στN\" -> 0.000021520778    |>   , \n\"IDS0502_220603_RAW_cal__sam_\" ->   <|    \"ζ\" -> 0.000000000000   ,  \"τ1\" -> 0.000000000000   ,  \"τS\" -> 0.000000000000   ,  \"τN\" -> 0.000000000000   ,  \"τC\" -> 0.000000000000   ,  \"κ0\" -> 0.000000000000   ,  \"mm1\" -> 0.000000000000   ,  \"mm2\" -> 0.000000000000   ,  \"mm3\" -> 0.000000000000   ,  \"T\" -> 0.620000000000   ,  \"B\" -> 8.000000000000   ,  \"θ\" -> 45.000000000000   ,  \"Reoff\" -> 0.000000000000   ,  \"Imoff\" -> 0.000000000000   ,  \"στ1\" -> 0.000000000000   ,  \"στS\" -> 0.000000000000   ,  \"στN\" -> 0.000000000000    |>   , \n\"IDS0503_220603_RAW_cal__ref_\" ->   <|    \"ζ\" -> 0.027095379561   ,  \"τ1\" -> 0.013653054815   ,  \"τS\" -> 0.022995805893   ,  \"τN\" -> 0.000444319703   ,  \"τC\" -> 0.002402226581   ,  \"κ0\" -> 0.000000005139   ,  \"mm1\" -> 0.000057649030   ,  \"mm2\" -> 0.013182559678   ,  \"mm3\" -> 0.026890317385   ,  \"T\" -> 0.820000000000   ,  \"B\" -> 8.000000000000   ,  \"θ\" -> 45.000000000000   ,  \"Reoff\" -> -959183.673469387459   ,  \"Imoff\" -> 0.000000000000   ,  \"στ1\" -> 0.001867148954   ,  \"στS\" -> 0.000121343744   ,  \"στN\" -> 0.000029055500    |>   , \n\"IDS0503_220603_RAW_cal__sam_\" ->   <|    \"ζ\" -> 0.000000000000   ,  \"τ1\" -> 0.000000000000   ,  \"τS\" -> 0.000000000000   ,  \"τN\" -> 0.000000000000   ,  \"τC\" -> 0.000000000000   ,  \"κ0\" -> 0.000000000000   ,  \"mm1\" -> 0.000000000000   ,  \"mm2\" -> 0.000000000000   ,  \"mm3\" -> 0.000000000000   ,  \"T\" -> 0.820000000000   ,  \"B\" -> 8.000000000000   ,  \"θ\" -> 45.000000000000   ,  \"Reoff\" -> 0.000000000000   ,  \"Imoff\" -> 0.000000000000   ,  \"στ1\" -> 0.000000000000   ,  \"στS\" -> 0.000000000000   ,  \"στN\" -> 0.000000000000    |>   , \n\"IDS0504_220603_RAW_cal__ref_\" ->   <|    \"ζ\" -> 0.022447798358   ,  \"τ1\" -> 0.013732237823   ,  \"τS\" -> 0.018577417913   ,  \"τN\" -> 0.000173926586   ,  \"τC\" -> 0.002459582749   ,  \"κ0\" -> 0.000000007201   ,  \"mm1\" -> 0.000047916077   ,  \"mm2\" -> 0.013432779765   ,  \"mm3\" -> 0.021883395630   ,  \"T\" -> 1.120000000000   ,  \"B\" -> 8.000000000000   ,  \"θ\" -> 45.000000000000   ,  \"Reoff\" -> -714285.714285713619   ,  \"Imoff\" -> 0.000000000000   ,  \"στ1\" -> 0.000607993232   ,  \"στS\" -> 0.000105526265   ,  \"στN\" -> 0.000003332790    |>   , \n\"IDS0504_220603_RAW_cal__sam_\" ->   <|    \"ζ\" -> 0.000000000000   ,  \"τ1\" -> 0.000000000000   ,  \"τS\" -> 0.000000000000   ,  \"τN\" -> 0.000000000000   ,  \"τC\" -> 0.000000000000   ,  \"κ0\" -> 0.000000000000   ,  \"mm1\" -> 0.000000000000   ,  \"mm2\" -> 0.000000000000   ,  \"mm3\" -> 0.000000000000   ,  \"T\" -> 1.120000000000   ,  \"B\" -> 8.000000000000   ,  \"θ\" -> 45.000000000000   ,  \"Reoff\" -> 0.000000000000   ,  \"Imoff\" -> 0.000000000000   ,  \"στ1\" -> 0.000000000000   ,  \"στS\" -> 0.000000000000   ,  \"στN\" -> 0.000000000000    |>   , \n\"IDS0505_220603_RAW_cal__ref_\" ->   <|    \"ζ\" -> 0.017603951649   ,  \"τ1\" -> 0.013742471601   ,  \"τS\" -> 0.012869162108   ,  \"τN\" -> 0.000062251305   ,  \"τC\" -> 0.002783258647   ,  \"κ0\" -> 0.000000012669   ,  \"mm1\" -> 0.000039808958   ,  \"mm2\" -> 0.013395445115   ,  \"mm3\" -> 0.016249533565   ,  \"T\" -> 1.900000000000   ,  \"B\" -> 8.000000000000   ,  \"θ\" -> 45.000000000000   ,  \"Reoff\" -> -322448.979591836221   ,  \"Imoff\" -> 0.000000000000   ,  \"στ1\" -> 0.000975208988   ,  \"στS\" -> 0.000083582947   ,  \"στN\" -> 0.000002846022    |>   , \n\"IDS0505_220603_RAW_cal__sam_\" ->   <|    \"ζ\" -> 0.000000000000   ,  \"τ1\" -> 0.000000000000   ,  \"τS\" -> 0.000000000000   ,  \"τN\" -> 0.000000000000   ,  \"τC\" -> 0.000000000000   ,  \"κ0\" -> 0.000000000000   ,  \"mm1\" -> 0.000000000000   ,  \"mm2\" -> 0.000000000000   ,  \"mm3\" -> 0.000000000000   ,  \"T\" -> 1.900000000000   ,  \"B\" -> 8.000000000000   ,  \"θ\" -> 45.000000000000   ,  \"Reoff\" -> 0.000000000000   ,  \"Imoff\" -> 0.000000000000   ,  \"στ1\" -> 0.000000000000   ,  \"στS\" -> 0.000000000000   ,  \"στN\" -> 0.000000000000    |>   , \n\"IDS0506_220603_RAW_cal__ref_\" ->   <|    \"ζ\" -> 0.017513535650   ,  \"τ1\" -> 0.013742433942   ,  \"τS\" -> 0.009294247030   ,  \"τN\" -> 0.000023643269   ,  \"τC\" -> 0.002563999230   ,  \"κ0\" -> 0.000000022469   ,  \"mm1\" -> 0.000034819598   ,  \"mm2\" -> 0.011836880672   ,  \"mm3\" -> 0.013915812404   ,  \"T\" -> 3.100000000000   ,  \"B\" -> 8.000000000000   ,  \"θ\" -> 45.000000000000   ,  \"Reoff\" -> -175510.204081632197   ,  \"Imoff\" -> 0.000000000000   ,  \"στ1\" -> 0.000768522779   ,  \"στS\" -> 0.000063413326   ,  \"στN\" -> 0.000000634158    |>   , \n\"IDS0506_220603_RAW_cal__sam_\" ->   <|    \"ζ\" -> 0.000000000000   ,  \"τ1\" -> 0.000000000000   ,  \"τS\" -> 0.000000000000   ,  \"τN\" -> 0.000000000000   ,  \"τC\" -> 0.000000000000   ,  \"κ0\" -> 0.000000000000   ,  \"mm1\" -> 0.000000000000   ,  \"mm2\" -> 0.000000000000   ,  \"mm3\" -> 0.000000000000   ,  \"T\" -> 3.100000000000   ,  \"B\" -> 8.000000000000   ,  \"θ\" -> 45.000000000000   ,  \"Reoff\" -> 0.000000000000   ,  \"Imoff\" -> 0.000000000000   ,  \"στ1\" -> 0.000000000000   ,  \"στS\" -> 0.000000000000   ,  \"στN\" -> 0.000000000000    |>   , \n\"IDS0508_220603_RAW_cal__ref_\" ->   <|    \"ζ\" -> 0.243281471751   ,  \"τ1\" -> 0.025048654847   ,  \"τS\" -> 0.062611130643   ,  \"τN\" -> 0.020042988527   ,  \"τC\" -> 0.000849297815   ,  \"κ0\" -> 0.000000000907   ,  \"mm1\" -> 0.000164736185   ,  \"mm2\" -> 0.017764187201   ,  \"mm3\" -> 0.110731364203   ,  \"T\" -> 0.200000000000   ,  \"B\" -> 6.000000000000   ,  \"θ\" -> 45.000000000000   ,  \"Reoff\" -> -40636734.693877548000   ,  \"Imoff\" -> 0.000000000000   ,  \"στ1\" -> 0.014234353727   ,  \"στS\" -> 0.004838976210   ,  \"στN\" -> 0.004976250052    |>   , \n\"IDS0508_220603_RAW_cal__sam_\" ->   <|    \"ζ\" -> 0.000000000000   ,  \"τ1\" -> 0.000000000000   ,  \"τS\" -> 0.000000000000   ,  \"τN\" -> 0.000000000000   ,  \"τC\" -> 0.000000000000   ,  \"κ0\" -> 0.000000000000   ,  \"mm1\" -> 0.000000000000   ,  \"mm2\" -> 0.000000000000   ,  \"mm3\" -> 0.000000000000   ,  \"T\" -> 0.200000000000   ,  \"B\" -> 6.000000000000   ,  \"θ\" -> 45.000000000000   ,  \"Reoff\" -> 0.000000000000   ,  \"Imoff\" -> 0.000000000000   ,  \"στ1\" -> 0.000000000000   ,  \"στS\" -> 0.000000000000   ,  \"στN\" -> 0.000000000000    |>   , \n\"IDS0509_220603_RAW_cal__ref_\" ->   <|    \"ζ\" -> 0.413507557358   ,  \"τ1\" -> 0.033675995603   ,  \"τS\" -> 0.093816108912   ,  \"τN\" -> 0.061390510422   ,  \"τC\" -> 0.000803159189   ,  \"κ0\" -> 0.000000000612   ,  \"mm1\" -> 0.000233947412   ,  \"mm2\" -> 0.019125451380   ,  \"mm3\" -> 0.234505485381   ,  \"T\" -> 0.150000000000   ,  \"B\" -> 6.000000000000   ,  \"θ\" -> 45.000000000000   ,  \"Reoff\" -> -88975510.204081654600   ,  \"Imoff\" -> 0.000000000000   ,  \"στ1\" -> 0.030359635336   ,  \"στS\" -> 0.022777334435   ,  \"στN\" -> 0.025753606266    |>   , \n\"IDS0509_220603_RAW_cal__sam_\" ->   <|    \"ζ\" -> 0.000000000000   ,  \"τ1\" -> 0.000000000000   ,  \"τS\" -> 0.000000000000   ,  \"τN\" -> 0.000000000000   ,  \"τC\" -> 0.000000000000   ,  \"κ0\" -> 0.000000000000   ,  \"mm1\" -> 0.000000000000   ,  \"mm2\" -> 0.000000000000   ,  \"mm3\" -> 0.000000000000   ,  \"T\" -> 0.150000000000   ,  \"B\" -> 6.000000000000   ,  \"θ\" -> 45.000000000000   ,  \"Reoff\" -> 0.000000000000   ,  \"Imoff\" -> 0.000000000000   ,  \"στ1\" -> 0.000000000000   ,  \"στS\" -> 0.000000000000   ,  \"στN\" -> 0.000000000000    |>   , \n\"IDS0510_220603_RAW_cal__ref_\" ->   <|    \"ζ\" -> 0.613284276562   ,  \"τ1\" -> 0.039588841090   ,  \"τS\" -> 0.126363579952   ,  \"τN\" -> 0.150529821612   ,  \"τC\" -> 0.000834158039   ,  \"κ0\" -> 0.000000000449   ,  \"mm1\" -> 0.000316290952   ,  \"mm2\" -> 0.017230786632   ,  \"mm3\" -> 0.469583692571   ,  \"T\" -> 0.120000000000   ,  \"B\" -> 6.000000000000   ,  \"θ\" -> 45.000000000000   ,  \"Reoff\" -> -183040816.326530635000   ,  \"Imoff\" -> 0.000000000000   ,  \"στ1\" -> 0.058972518993   ,  \"στS\" -> 0.069910296081   ,  \"στN\" -> 0.097464298744    |>   , \n\"IDS0510_220603_RAW_cal__sam_\" ->   <|    \"ζ\" -> 0.000000000000   ,  \"τ1\" -> 0.000000000000   ,  \"τS\" -> 0.000000000000   ,  \"τN\" -> 0.000000000000   ,  \"τC\" -> 0.000000000000   ,  \"κ0\" -> 0.000000000000   ,  \"mm1\" -> 0.000000000000   ,  \"mm2\" -> 0.000000000000   ,  \"mm3\" -> 0.000000000000   ,  \"T\" -> 0.120000000000   ,  \"B\" -> 6.000000000000   ,  \"θ\" -> 45.000000000000   ,  \"Reoff\" -> 0.000000000000   ,  \"Imoff\" -> 0.000000000000   ,  \"στ1\" -> 0.000000000000   ,  \"στS\" -> 0.000000000000   ,  \"στN\" -> 0.000000000000    |>   , \n\"IDS0511_220604_RAW_cal__ref_\" ->   <|    \"ζ\" -> 0.330310083388   ,  \"τ1\" -> 0.030298910704   ,  \"τS\" -> 0.075236256272   ,  \"τN\" -> 0.040258490760   ,  \"τC\" -> 0.000782924983   ,  \"κ0\" -> 0.000000000728   ,  \"mm1\" -> 0.000193254303   ,  \"mm2\" -> 0.018356930637   ,  \"mm3\" -> 0.166175477301   ,  \"T\" -> 0.170000000000   ,  \"B\" -> 6.000000000000   ,  \"θ\" -> 45.000000000000   ,  \"Reoff\" -> -64436734.693877577800   ,  \"Imoff\" -> 0.000000000000   ,  \"στ1\" -> 0.014626951982   ,  \"στS\" -> 0.008056203133   ,  \"στN\" -> 0.008938953770    |>   , \n\"IDS0511_220604_RAW_cal__sam_\" ->   <|    \"ζ\" -> 0.000000000000   ,  \"τ1\" -> 0.000000000000   ,  \"τS\" -> 0.000000000000   ,  \"τN\" -> 0.000000000000   ,  \"τC\" -> 0.000000000000   ,  \"κ0\" -> 0.000000000000   ,  \"mm1\" -> 0.000000000000   ,  \"mm2\" -> 0.000000000000   ,  \"mm3\" -> 0.000000000000   ,  \"T\" -> 0.170000000000   ,  \"B\" -> 6.000000000000   ,  \"θ\" -> 45.000000000000   ,  \"Reoff\" -> 0.000000000000   ,  \"Imoff\" -> 0.000000000000   ,  \"στ1\" -> 0.000000000000   ,  \"στS\" -> 0.000000000000   ,  \"στN\" -> 0.000000000000    |>   , \n\"IDS0512_220604_RAW_cal__ref_\" ->   <|    \"ζ\" -> 0.157633362112   ,  \"τ1\" -> 0.020861334985   ,  \"τS\" -> 0.051508696686   ,  \"τN\" -> 0.008332770174   ,  \"τC\" -> 0.001009053466   ,  \"κ0\" -> 0.000000001248   ,  \"mm1\" -> 0.000135415312   ,  \"mm2\" -> 0.017070380875   ,  \"mm3\" -> 0.073939070739   ,  \"T\" -> 0.250000000000   ,  \"B\" -> 6.000000000000   ,  \"θ\" -> 45.000000000000   ,  \"Reoff\" -> -16726530.612244904000   ,  \"Imoff\" -> 0.000000000000   ,  \"στ1\" -> 0.019204175583   ,  
